vi "GoBang_RemoveStonesFromLine.vi"(1 "line with 4 elements in":u8[](array[numeric])=[0, 0, 0, 0, 0]) -> (0 "line with 4 elements out":u8[](array[numeric]))   [LabVIEW 2014, in "GoBang.lvlib"]
uses:
  GoBang.lvlib
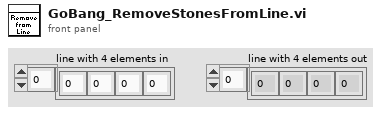
[diagram p1: front panel]
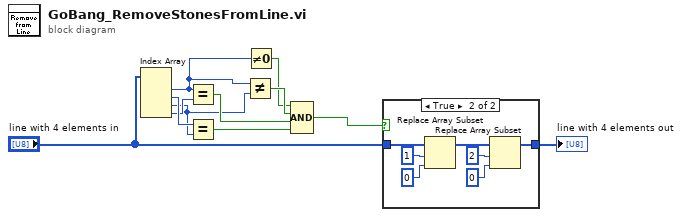
[diagram p0: block diagram]
diagram:
  n1 = Index Array(array="line with 4 elements in") -> (element #1=w2:u8, element #2=w6:u8, element #3=w3:u8, element #4=w5:u8)  [unwired: 4 in]
  n2 = Equal?(x=w2, y=w5) -> (x = y?=w11:bool)
  n3 = Equal?(x=w6, y=w3) -> (x = y?=w10:bool)
  n4 = Not Equal?(x=w2, y=w3) -> (x != y?=w4:bool)
  n5 = Not Equal To 0?(x=w2) -> (x != 0?=w1:bool)
  n6 = Compound Arithmetic op=AND(w1, w4, w11, w10) -> (w9:bool)
  n7 = case shown="True" w9 {
    tunnel: "line with 4 elements in" -> [w12 w19]
    tunnel: [w12 w17] -> w7
    frame False {
    }
    frame True {
      n8 = Replace Array Subset(array=w19, new element=u8 0 ("new element/subarray"), index=1) -> (w18:u8[])
      n9 = Replace Array Subset(array=w18, new element=u8 0 ("new element/subarray"), index=2) -> (w17:u8[])
    }
  }
  "line with 4 elements out" <- w7
